vi "ExReadR3BFileHeader.vi"(1 "error in (no error)":errorcluster) -> (0 "error out":errorcluster)   [LabVIEW 2010]
panel:
  out "End Tic Count":u64
  out "Start Tic Count":u64
  out "End Date/Time (UTCl) Num":u32
  out "End Date/Time (Local) Num":u32
  out "End Date/Time (UTC)":string
  out "End Date/Time (Local)":string
  out "Start Date/Time (UTCl) Num":u32
  out "Start Date/Time (Local) Num":u32
  out "Date/Time (UTC)":string
  out "Date/Time (Local)":string
  out "File Version":u32
  out "Data Type":u32
  out "Number of Frames":u32
  out "Y Size":u32
  out "X Size":u32
  in  "Full File Name":path
  in  "FileType":u32=67633152
  # "ExReadR3BFileHeader.vi\nThis VI will use read information stored in the file header and display it."
  # "File Types:\nSPE = 67371008\nTIF  = 67174400\nR3B = 67633152\nPMI = 67436544"
  # "Browse match pattern is set to *.r3b.  Modify this if different file type is needed."
  # "START"
  # "Data Types:\n1 = 8 bit signed char\n2 = 16 bit signed integer\n3 = 32 bit signed integer\n4 = 32 bit float\n5 = 64 bit float\n6 = 8 bit unsigned char\n7 = 16 bit unsigned integer\n8 = 32 bit unsigned integer"
  # "END"
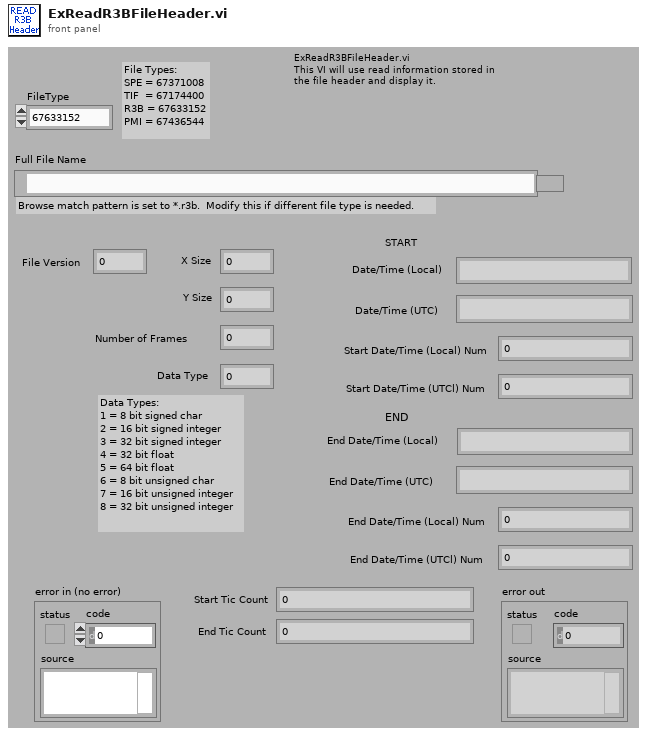
[diagram p1: front panel]
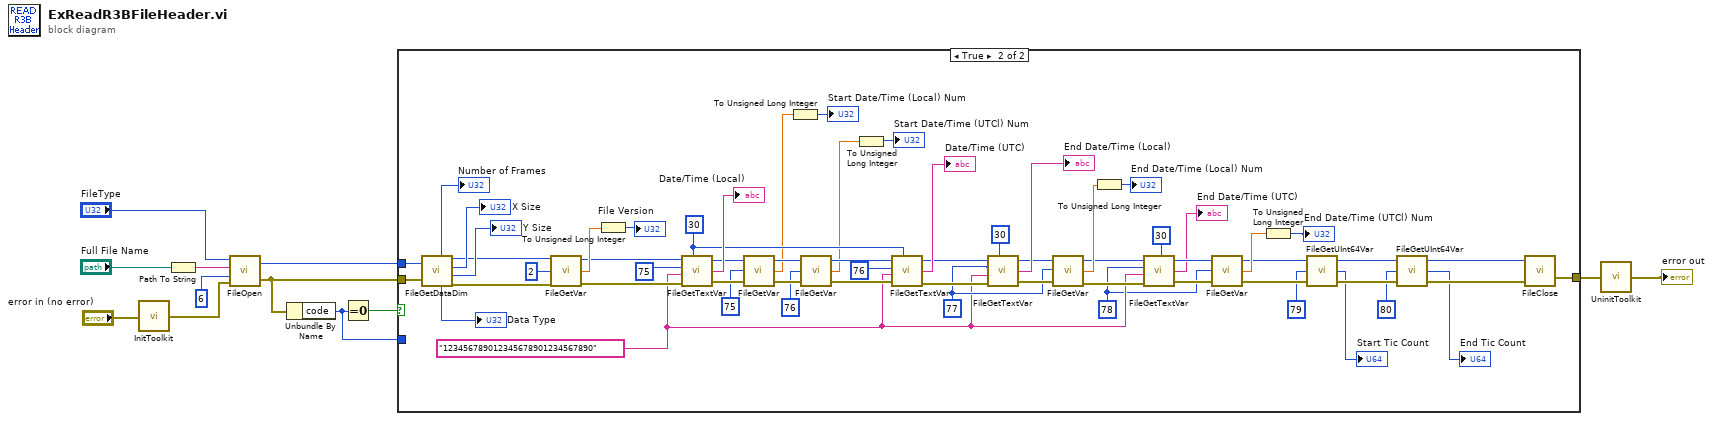
[diagram p0: block diagram]
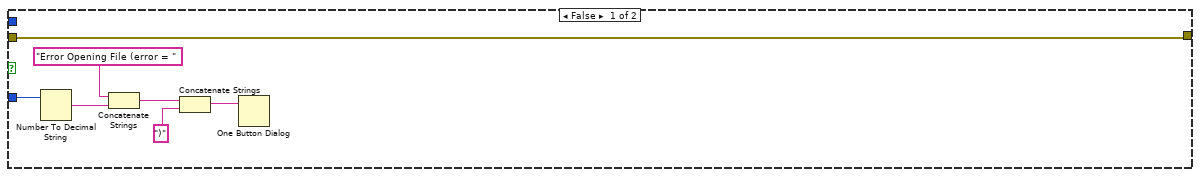
[diagram p2: hidden frame]
diagram:
  n1 = call <userlib>:"InitToolkit.vi"("error in"="error in (no error)") -> ("error out"=w3:errorcluster)
  n2 = Path To String(path="Full File Name") -> (string=w10:string)
  n3 = call <userlib>:"FileOpen.vi"("error in"=w3, "File Operations"=6, "FileName"=w10, "File Type"="FileType") -> ("error out"=w7:errorcluster, "File Handle"=w6:u32)
  n4 = Unbundle By Name(w7) -> ("code"=w5:i32)
  n5 = Equal To 0?(x=w5) -> (x = 0?=w8:bool)
  n6 = case shown="True" w8 {
    tunnel: w7 -> [w13 w79]
    tunnel: w6 -> [_ w78]
    tunnel: w5 -> [w19 _]
    tunnel: [w13 w61] -> w2
    frame False {
      n7 = Number To Decimal String(number=w19) -> (decimal integer string=w18:string)  [unwired: 1 in]
      n8 = Concatenate Strings("Error Opening File (error = ", w18) -> (w16:string)
      n9 = Concatenate Strings(w16, ")") -> (w14:string)
      n10 = One Button Dialog(message=w14) -> ()  [unwired: 1 in, 1 out]
    }
    frame True {
      w32 = 78
      w42 = 77
      w37 = "123456789012345678901234567890"
      w64 = 30
      n11 = call <userlib>:"FileGetDataDim.vi"("File Handle"=w78, "error in"=w79) -> ("Number of Frames"=→"Number of Frames":u32, "Data Type"=→"Data Type":u32, "File Handle"=w72:u32, "X dim"=→"X Size":u32, "Y dim"=→"Y Size":u32, "error out"=w73:errorcluster)
      n12 = call <userlib>:"FileGetVar.vi"("error in"=w73, "Parameter ID"=2, "File Handle"=w72) -> ("error out"=w68:errorcluster, "Value"=w70:dbl, "File Handle"=w67:u32)
      n13 = To Unsigned Long Integer(number=w70) -> (unsigned 32bit integer=→"File Version":u32)
      n14 = call <userlib>:"FileGetTextVar.vi"("File Handle"=w67, "Parameter ID"=75, "User Text Buffer"=w37, "error in"=w68, "Text Buffer Size"=w64) -> ("File Handle"=w57:u32, "Text Value Returned"=→"Date/Time (Local)":string, "error out"=w60:errorcluster)
      n15 = call <userlib>:"FileGetVar.vi"("error in"=w60, "Parameter ID"=75, "File Handle"=w57) -> ("error out"=w59:errorcluster, "Value"=w53:dbl, "File Handle"=w56:u32)
      n16 = To Unsigned Long Integer(number=w53) -> (unsigned 32bit integer=→"Start Date/Time (Local) Num":u32)
      n17 = call <userlib>:"FileGetVar.vi"("error in"=w59, "Parameter ID"=76, "File Handle"=w56) -> ("error out"=w58:errorcluster, "Value"=w50:dbl, "File Handle"=w55:u32)
      n18 = To Unsigned Long Integer(number=w50) -> (unsigned 32bit integer=→"Start Date/Time (UTCl) Num":u32)
      n19 = call <userlib>:"FileGetTextVar.vi"("File Handle"=w55, "Parameter ID"=76, "User Text Buffer"=w37, "error in"=w58, "Text Buffer Size"=w64) -> ("File Handle"=w48:u32, "Text Value Returned"=→"Date/Time (UTC)":string, "error out"=w47:errorcluster)
      n20 = call <userlib>:"FileGetTextVar.vi"("File Handle"=w48, "Parameter ID"=w42, "User Text Buffer"=w37, "error in"=w47, "Text Buffer Size"=30) -> ("File Handle"=w44:u32, "Text Value Returned"=→"End Date/Time (Local)":string, "error out"=w43:errorcluster)
      n21 = call <userlib>:"FileGetVar.vi"("error in"=w43, "Parameter ID"=w42, "File Handle"=w44) -> ("error out"=w38:errorcluster, "Value"=w40:dbl, "File Handle"=w39:u32)
      n22 = To Unsigned Long Integer(number=w40) -> (unsigned 32bit integer=→"End Date/Time (Local) Num":u32)
      n23 = call <userlib>:"FileGetTextVar.vi"("File Handle"=w39, "Parameter ID"=w32, "User Text Buffer"=w37, "error in"=w38, "Text Buffer Size"=30) -> ("File Handle"=w34:u32, "Text Value Returned"=→"End Date/Time (UTC)":string, "error out"=w35:errorcluster)
      n24 = call <userlib>:"FileGetVar.vi"("error in"=w35, "Parameter ID"=w32, "File Handle"=w34) -> ("error out"=w30:errorcluster, "Value"=w29:dbl, "File Handle"=w26:u32)
      n25 = To Unsigned Long Integer(number=w29) -> (unsigned 32bit integer=→"End Date/Time (UTCl) Num":u32)
      n26 = call <userlib>:"FileGetUInt64Var.vi"("error in"=w30, "Parameter ID"=79, "File Handle"=w26) -> ("error out"=w28:errorcluster, "Value"=→"Start Tic Count":u64, "File Handle"=w25:u32)
      n27 = call <userlib>:"FileGetUInt64Var.vi"("error in"=w28, "Parameter ID"=80, "File Handle"=w25) -> ("error out"=w27:errorcluster, "Value"=→"End Tic Count":u64, "File Handle"=w24:u32)
      n28 = call <userlib>:"FileClose.vi"("error in"=w27, "File Handle"=w24) -> ("error out"=w61:errorcluster)
    }
  }
  n29 = call <userlib>:"UninitToolkit.vi"("error in"=w2) -> ("error out"=→"error out":errorcluster)
